vi "Illumination_Interp_2015LED.vi"(0 "LEDAD Port":refnum<visa-resource-name>="COM7", 1 "Mode":T1, 7 "Illumination Desired":dbl(slide) scale=0.0..100.0, 9 "Enable LED":u8(slide) scale=0.0..31.0, 11 "error in (no error)":errorcluster, 13 "Calibration File":path) -> (4 "LEDAD Port out":refnum<visa-resource-name>, 8 "Intensity":dbl format="%#_4g", 10 "Variance":dbl format="%#_4g", 15 "error out":errorcluster)   [LabVIEW 2010]
uses:
  Projects/2015 Multiport/Type Definitions/CamMode_TypeDef.ctl
  <vilib>/Utility/file.llb/Read From Spreadsheet File (DBL).vi
panel:
  # "%"
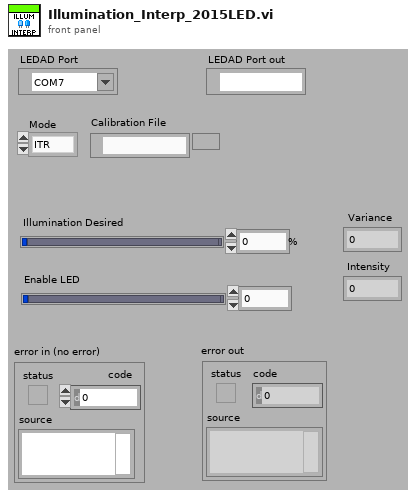
[diagram p1: front panel]
types:
  T1 = typedef "CamMode_TypeDef.ctl" = enum8{"ITR", "CDS", "IWR", "sCMOS"}
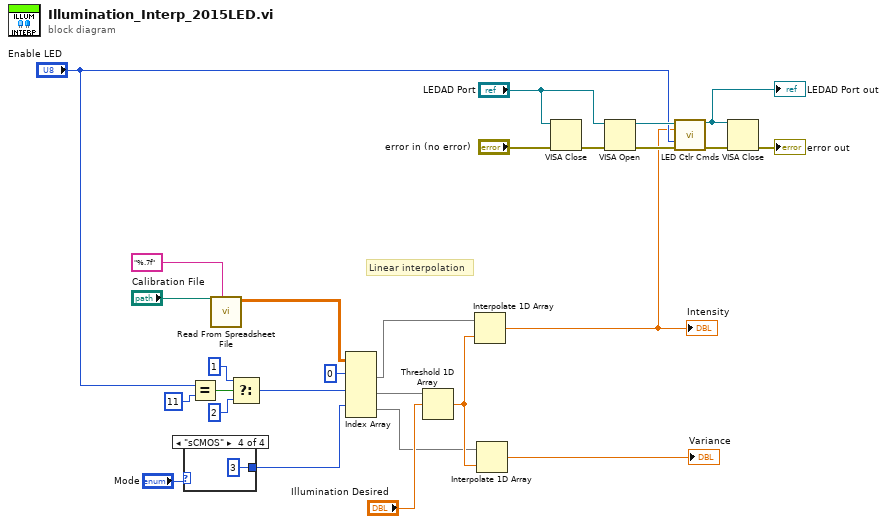
[diagram p0: block diagram]
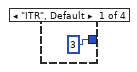
[diagram p2: hidden frame]
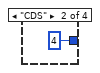
[diagram p3: hidden frame]
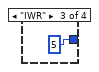
[diagram p4: hidden frame]
diagram:
  # "Linear interpolation"
  n1 = case shown="\"sCMOS\"" "Mode" {
    tunnel: [3 ("index") 4 ("index") 5 ("index") 3 ("index")] -> w2
    frame "ITR", Default {
    }
    frame "CDS" {
    }
    frame "IWR" {
    }
    frame "sCMOS" {
    }
  }
  n2 = Equal?(x="Enable LED", y=u8 11) -> (x = y?=w12:bool)
  n3 = call-poly <vilib>:"Read From Spreadsheet File.vi"("format (%.3f)"="%.7f", "file path (dialog if empty)"="Calibration File") -> ("all rows"=w15:dbl[][])  [unwired: 5 in, 4 out]
  n4 = Select(t=1 ("index (row)"), s=w12, f=2) -> (s? t:f=w6:i32)
  n5 = Index Array(array=w15, index (row) #1=0 ("index (row)"), index (row) #2=w6, index (row) #3=w2) -> (element #1=w4:dbl[], element #2=w5:dbl[], element #3=w1:dbl[])  [unwired: 3 in]
  n6 = Threshold 1D Array(2:"Illumination Desired", 3:w5) -> (0:w8:dbl)  [unwired: 1 in]
  n7 = Interpolate 1D Array(1:w8, 2:w4) -> (0:w9:dbl)
  "Intensity" <- w9
  n8 = Interpolate 1D Array(1:w8, 2:w1) -> (0:→"Variance":dbl)
  n9 = VISA Close(VISA resource name="LEDAD Port", error in (no error)="error in (no error)") -> (error out=w20:errorcluster)
  n10 = VISA Open(error in (no error)=w20, VISA resource name="LEDAD Port") -> (VISA resource name=w21:refnum<visa-resource-name>, error out=w25:errorcluster)  [unwired: 3 in]
  n11 = call "LED Ctlr Cmds.vi"("VISA session"=w21, "Intensity"=w9, "Enable"="Enable LED", "error in (no error)"=w25) -> ("VISA session out"=w22:refnum<visa-resource-name>, "error out"=w24:errorcluster)  [unwired: 7 in, 3 out]
  "LEDAD Port out" <- w22
  n12 = VISA Close(VISA resource name=w22, error in (no error)=w24) -> (error out=→"error out":errorcluster)
